vi "Configure Interpolation [I] Core.vi"(8 "error in (no error)":errorcluster, 10 "interpolation":i32(ring)=1 items=["No Interpolation"=1, "sin(x)/x"=2, "Linear Interpolation"=3], 11 "CS++Scope":refnum<class "CS++Scope.lvclass">) -> (0 "error out":errorcluster, 3 "CS++Scope out":refnum<class "CS++Scope.lvclass">)   [LabVIEW 2016, in "CS++Scope.lvlib" / "CS++Scope.lvclass"]
doc: "This VI configures the interpolation method the oscilloscope uses when it cannot sample a voltage for a point in the waveform record. \n\nNotes:\n\n(1) This VI is part of the miscellaneous [*] extension group."
uses:
  CS++Scope.lvclass
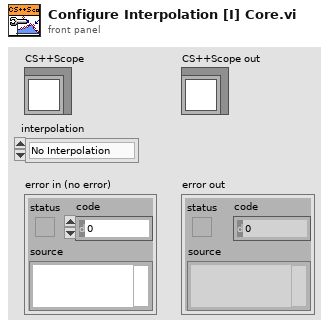
[diagram p1: front panel]
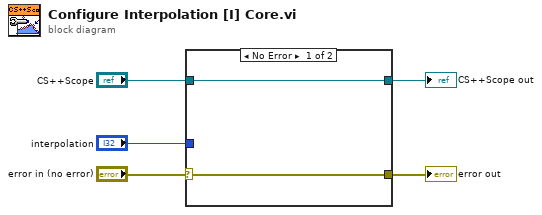
[diagram p0: block diagram]
diagram:
  n1 = case shown="No Error" "error in (no error)" {
    selector: "error in (no error)" -> [w6 w9]
    tunnel: [w6 w9] -> w4
    tunnel: [w7 w8] -> w2
    tunnel: "CS++Scope" -> [w7 w8]
    tunnel: "interpolation" -> [_ _]
    frame No Error {
    }
    frame Error {
    }
  }
  "error out" <- w4
  "CS++Scope out" <- w2
